vi "Finish.vi"   [LabVIEW 2014]
doc: "This VI is called just before exiting. It is expected to close I/O refnum, save collected data, etc."
uses:
  Robot Global ref.vi
types:
  T1 = typedef "Robot Global ref.ctl" = cluster{"Joysticks":cluster{"OpJoystickRef":T2, "DriveJoystickRef":T2, "DriveJoystickRef2":T2}, "Drive Motors Ref":cluster{"RobotDriveDevRef":T4}, "Ultrasonic":cluster{"AIDeviceRef":T12}, "Shifters":cluster{"SolenoidDevRef":T15}, "Gyro":cluster{"GyroDevRef":T18}, "Acquistion sensor":cluster{"HighDIO":T19, "Acquisition Bottom1":T19, "Acquisition Top":T19, "Acquisition Bottom2":T19}, "Motors":cluster{"AcqMotorRef":T5, "ShooterMotorRef":T5, "AcqshoulderControlDeviceRef":T5, "LatchControlDeviceRef":T5}, "Servos":cluster{"Winch Servo ":T21, "TrajectorycontrolDeviceRef":T21}, "Shooter Latch Sensors":cluster{"Shooter Latch Sensor Top":T19, "Shooter Latch Sensor Bottom":T19}, "Ring light relay":cluster{"RelayDevRef":T22}}
  T2 = typedef "WPI_JoystickDevRef.ctl" = cluster{"Device":T3}
  T3 = typedef "WPI_JoystickDeviceEnum.ctl" = enum16{"USB 0", "USB 1", "USB 2", "USB 3", "USB 4", "USB 5"}
  T4 = typedef "WPI_RobotDriveDevRef.ctl" = cluster{"DevStatus":errorcluster, "Motors[]":T5[], "Square Inputs":bool, "Max Output":dbl}
  T5 = typedef "WPI_MotorControlDeviceRef.ctl" = cluster{"DeviceStatus":errorcluster, "Type":enum16{"PWM", "CAN"}, "PWM":cluster{"Digital Module":T6, "PWM Channel":T7, "DeadBand":T8}, "CAN":cluster{"Device Number":u8, "Control Mode":T9, "Semaphore":T10, "Max Vout":dbl}, "Invert":bool, "TransformRef":T11, "InvTransformRef":T11}
  T6 = typedef "FPGA_TypedefDigitalModule.ctl" = enum16{"Digital Module 1", "Digital Module 2"}
  T7 = typedef "FPGA_DIOPWMChannel.ctl" = enum8{"PWM 1", "PWM 2", "PWM 3", "PWM 4", "PWM 5", "PWM 6", "PWM 7", "PWM 8", "PWM 9", "PWM 10", "Invalid"}
  T8 = typedef "WPI_PWMDeadband.ctl" = cluster{"Name":string, "maxPositivePwm":i32, "minPositivePwm":i32, "centerPwm":i32, "maxNegativePwm":i32, "minNegativePwm":i32, "angularRange":u16}
  T9 = typedef "WPI_CANJaguar_ControlMode.ctl" = enum8{"Percent VBus", "Current", "Speed", "Position", "Voltage"}
  T10 = typedef "Semaphore RefNum" = refnum<k1>
  T11 = typedef "WPI_PWMTransform_ConPane.ctl" = refnum<vi>
  T12 = typedef "WPI_AnalogChannelDevRef.ctl" = cluster{"DevStatus":errorcluster, "Analog Module":T13, "Analog Channel":T14}
  T13 = typedef "FPGA_TypedefAnalogModule.ctl" = enum16{"Analog Module 1", "Analog Module 2"}
  T14 = typedef "FPGA_AIChannel.ctl" = enum8{"AI 1", "AI 2", "AI 3", "AI 4", "AI 5", "AI 6", "AI 7", "AI 8", "Invalid"}
  T15 = typedef "WPI_SolenoidDevRef.ctl" = cluster{"DevStatus":errorcluster, "Solenoid Module":T16, "Forward Solenoid Channel":T17, "Reverse Solenoid Channel":T17}
  T16 = typedef "FPGA_TypedefSolenoidModule.ctl" = enum16{"Solenoid Module 1", "Solenoid Module 2"}
  T17 = typedef "WPI_SolenoidChannel.ctl" = enum8{"Solenoid 1", "Solenoid 2", "Solenoid 3", "Solenoid 4", "Solenoid 5", "Solenoid 6", "Solenoid 7", "Solenoid 8", "Invalid"}
  T18 = typedef "WPI_GyroDevRef.ctl" = cluster{"DevStatus":errorcluster, "Analog Module":T13, "Analog Channel":T14, "Offset":dbl, "Gain (VoltsPerDegree/Second)":dbl}
  T19 = typedef "WPI_DigitalInputDevRef.ctl" = cluster{"DevStatus":errorcluster, "DIO Channel":T20, "Digital Module":T6}
  T20 = typedef "FPGA_DIOChannel.ctl" = enum8{"DIO 1", "DIO 2", "DIO 3", "DIO 4", "DIO 5", "DIO 6", "DIO 7", "DIO 8", "DIO 9", "DIO 10", "DIO 11", "DIO 12", "DIO 13", "DIO 14", "Invalid"}
  T21 = typedef "WPI_ServoDeviceRef.ctl" = cluster{"DeviceStatus":errorcluster, "Digital Module":T6, "PWM Channel":T7, "DeadBand":T8}
  T22 = typedef "WPI_RelayDevRef.ctl" = cluster{"DevStatus":errorcluster, "Relay Channel":T23, "Digital Module":T6, "Relay Direction":T24}
  T23 = typedef "FPGA_DIORelayChannel.ctl" = enum8{"Relay 1", "Relay 2", "Relay 3", "Relay 4", "Relay 5", "Relay 6", "Relay 7", "Relay 8", "Invalid"}
  T24 = typedef "WPI_RelayDirection.ctl" = enum16{"Both directions", "Forward only", "Reverse only"}
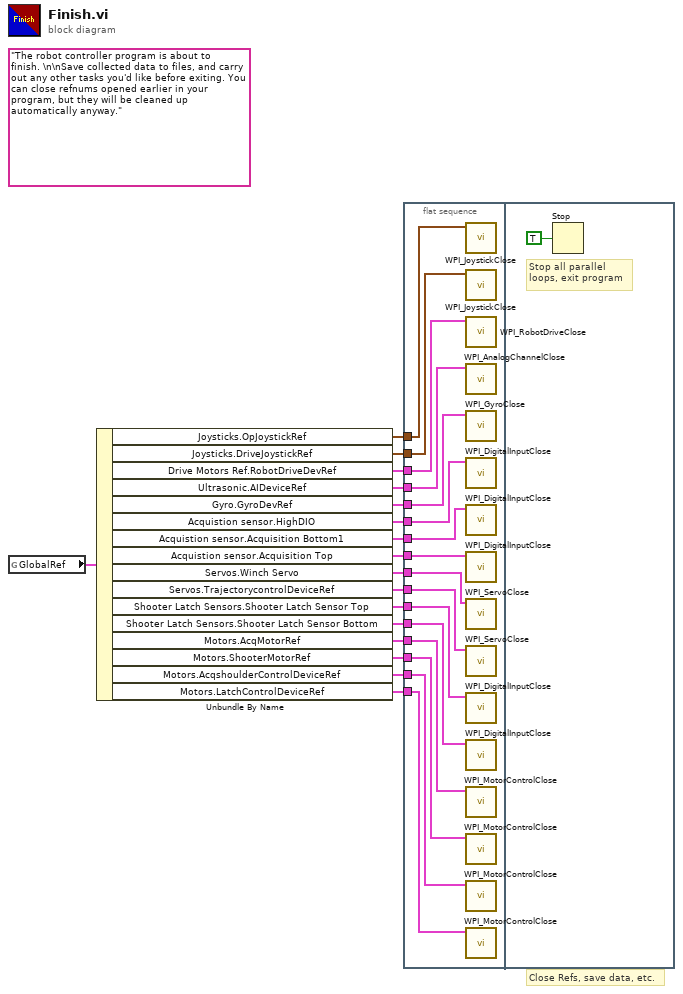
[diagram p0: block diagram]
diagram:
  (unwired) "The robot controller program is about to finish. \n\nSave collected data to files, and carry out any other tasks you'd like before exiting. You can close refnums opened earlier in your program, but they will be cleaned up automatically anyway."
  # "Close Refs, save data, etc."
  n1 = global read "Robot Global ref.vi" "GlobalRef"() -> (w17:T1)
  n2 = Unbundle By Name(w17) -> ("Joysticks.OpJoystickRef"=w14:T2, "Joysticks.DriveJoystickRef"=w15:T2, "Drive Motors Ref.RobotDriveDevRef"=w16:T4, "Ultrasonic.AIDeviceRef"=w13:T12, "Gyro.GyroDevRef"=w12:T18, "Acquistion sensor.HighDIO"=w11:T19, "Acquistion sensor.Acquisition Bottom1"=w10:T19, "Acquistion sensor.Acquisition Top"=w9:T19, "Servos.Winch Servo"=w8:T21, "Servos.TrajectorycontrolDeviceRef"=w7:T21, "Shooter Latch Sensors.Shooter Latch Sensor Top"=w6:T19, "Shooter Latch Sensors.Shooter Latch Sensor Bottom"=w5:T19, "Motors.AcqMotorRef"=w4:T5, "Motors.ShooterMotorRef"=w3:T5, "Motors.AcqshoulderControlDeviceRef"=w2:T5, "Motors.LatchControlDeviceRef"=w1:T5)
  n3 = flat-sequence {
    tunnel: w16 -> [w33]
    tunnel: w15 -> [w32]
    tunnel: w14 -> [w31]
    tunnel: w13 -> [w30]
    tunnel: w12 -> [w29]
    tunnel: w11 -> [w28]
    tunnel: w10 -> [w27]
    tunnel: w9 -> [w26]
    tunnel: w8 -> [w25]
    tunnel: w7 -> [w24]
    tunnel: w6 -> [w23]
    tunnel: w5 -> [w22]
    tunnel: w4 -> [w21]
    tunnel: w3 -> [w20]
    tunnel: w2 -> [w19]
    tunnel: w1 -> [w18]
    frame #0 {
      n4 = call <vilib>:"WPI_JoystickClose.vi"("JoystickDevRef"=w31) -> ()  [unwired: 11 out]
      n5 = call <vilib>:"WPI_JoystickClose.vi"("JoystickDevRef"=w32) -> ()  [unwired: 11 out]
      n6 = call <vilib>:"WPI_RobotDriveClose.vi"("RobotDriveDevRef"=w33) -> ()  [unwired: 1 in, 10 out]
      n7 = call <vilib>:"WPI_AnalogChannelClose.vi"("AIDeviceRef"=w30) -> ()  [unwired: 10 in, 1 out]
      n8 = call <vilib>:"WPI_GyroClose.vi"("GyroDevRef"=w29) -> ()  [unwired: 10 in, 1 out]
      n9 = call <vilib>:"WPI_DigitalInputClose.vi"("DigitalInputDevRef"=w28) -> ()  [unwired: 10 in, 1 out]
      n10 = call <vilib>:"WPI_DigitalInputClose.vi"("DigitalInputDevRef"=w27) -> ()  [unwired: 10 in, 1 out]
      n11 = call <vilib>:"WPI_DigitalInputClose.vi"("DigitalInputDevRef"=w26) -> ()  [unwired: 10 in, 1 out]
      n12 = call <vilib>:"WPI_ServoClose.vi"("MotorControlDevRef"=w25) -> ()  [unwired: 10 in, 1 out]
      n13 = call <vilib>:"WPI_ServoClose.vi"("MotorControlDevRef"=w24) -> ()  [unwired: 10 in, 1 out]
      n14 = call <vilib>:"WPI_DigitalInputClose.vi"("DigitalInputDevRef"=w23) -> ()  [unwired: 10 in, 1 out]
      n15 = call <vilib>:"WPI_DigitalInputClose.vi"("DigitalInputDevRef"=w22) -> ()  [unwired: 10 in, 1 out]
      n16 = call <vilib>:"WPI_MotorControlClose.vi"("MotorControlDevRef"=w21) -> ()  [unwired: 10 in, 1 out]
      n17 = call <vilib>:"WPI_MotorControlClose.vi"("MotorControlDevRef"=w20) -> ()  [unwired: 10 in, 1 out]
      n18 = call <vilib>:"WPI_MotorControlClose.vi"("MotorControlDevRef"=w19) -> ()  [unwired: 10 in, 1 out]
      n19 = call <vilib>:"WPI_MotorControlClose.vi"("MotorControlDevRef"=w18) -> ()  [unwired: 10 in, 1 out]
    }
    frame #1 {
      # "Stop all parallel\nloops, exit program"
      n20 = Stop(stop? (T)=TRUE ("Quit")) -> ()
    }
  }
